vi "contour_levels_to_list.vi"(6 "Anchored Num":dbl, 7 "Mode":enum16{"Levels", "Intervals", "Level List"}(ring), 8 "Anchored at":bool, 9 "Min Max":T1, 10 "Levels/Int":sgl caption="Levels", 11 "Dimension":u16(ring) caption="Axis" items=["X", "Y", "Z"]) -> (3 "Item Names":string[](array[string]))   [LabVIEW 2020, in "3DPC_SurfacePlot.xctl"]
uses:
  <vilib>/Native 3D Graph/xcontrol/3DPC_SurfacePlot.xctl
  <vilib>/Native 3D Graph/typedefs/range_cluster.ctl
  <vilib>/Native 3D Graph/typedefs/min_max.ctl
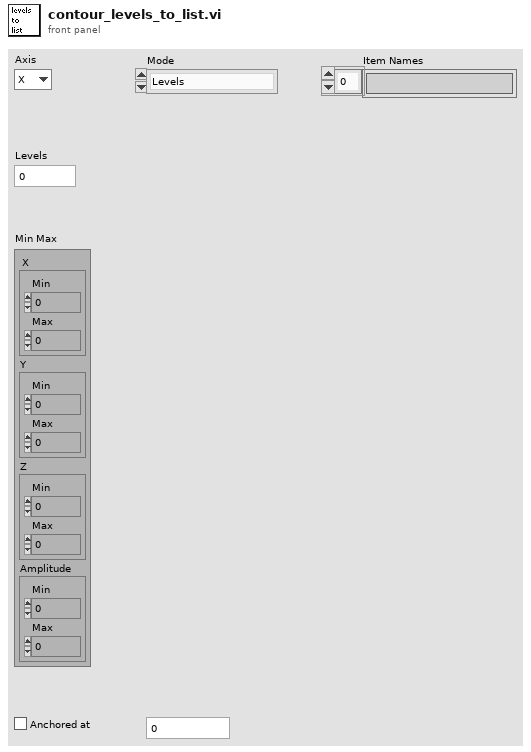
[diagram p1: front panel]
types:
  T1 = typedef "3DPC_SurfacePlot.xctl/range_cluster.ctl" = cluster{"X":T2, "Y":T2, "Z":T2, "Amplitude":T2}
  T2 = typedef "3DPC_SurfacePlot.xctl/min_max.ctl" = cluster{"Min":sgl, "Max":sgl}
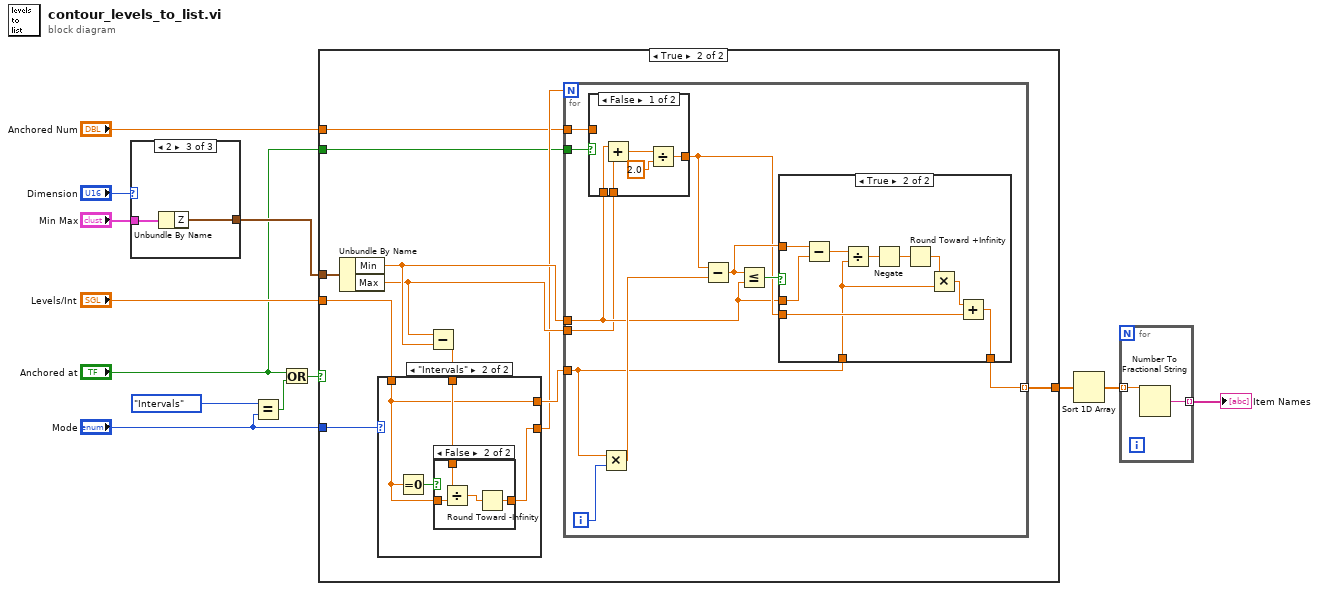
[diagram p0: block diagram]
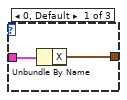
[diagram p2: hidden frame]
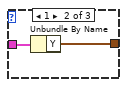
[diagram p3: hidden frame]
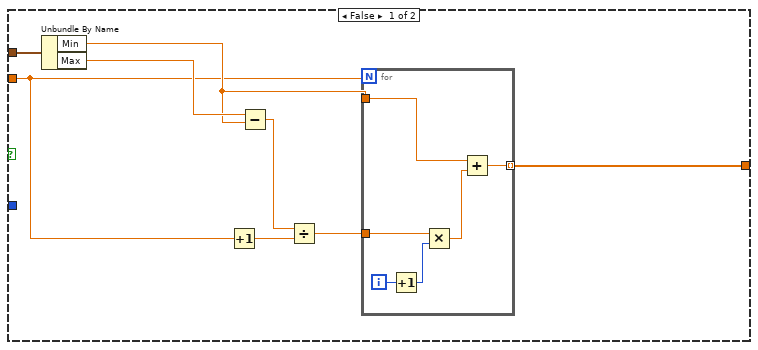
[diagram p4: hidden frame]
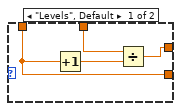
[diagram p5: hidden frame]
diagram:
  n1 = case shown="2" "Dimension" {
    tunnel: "Min Max" -> [w15 w17 w19]
    tunnel: [w14 w16 w18] -> w10
    frame 0, Default {
      n2 = Unbundle By Name(w15) -> ("X"=w14:T2)
    }
    frame 1 {
      n3 = Unbundle By Name(w17) -> ("Y"=w16:T2)
    }
    frame 2 {
      n4 = Unbundle By Name(w19) -> ("Z"=w18:T2)
    }
  }
  n5 = Equal?(x=enum16{"Levels", "Intervals", "Level List"}."Intervals" ("Mode"), y="Mode") -> (x = y?=w6:bool)
  n6 = Or(x="Anchored at", y=w6) -> (x .or. y?=w5:bool)
  n7 = case shown="True" w5 {
    tunnel: "Levels/Int" -> [w21 w40]
    tunnel: w10 -> [w27 w44]
    tunnel: [w22 w38] -> w8
    tunnel: "Mode" -> [_ w36]
    tunnel: "Anchored at" -> [_ w35]
    tunnel: "Anchored Num" -> [_ w34]
    frame False {
      n8 = Unbundle By Name(w27) -> ("Min"=w25:sgl, "Max"=w26:sgl)
      n9 = Increment(x=w21) -> (x+1=w20:sgl)
      n10 = Subtract(x=w26, y=w25) -> (x-y=w24:sgl)
      n11 = Divide(x=w24, y=w20) -> (x/y=w23:sgl)
      n12 = for {
        N: w21 -> [_]
        tunnel: w25 -> [w32]
        tunnel: w23 -> [w33]
        tunnel: [w28] -> w22 mode=indexing
        i -> [w30]
        n13 = Increment(x=w30) -> (x+1=w29:i32)
        n14 = Multiply(x=w33, y=w29) -> (x*y=w31:sgl)
        n15 = Add(x=w32, y=w31) -> (x+y=w28:sgl)
      }
    }
    frame True {
      n16 = Unbundle By Name(w44) -> ("Min"=w43:sgl, "Max"=w39:sgl)
      n17 = Subtract(x=w39, y=w43) -> (x-y=w42:sgl)
      n18 = case shown="\"Intervals\"" w36 {
        tunnel: w42 -> [w48 w52]
        tunnel: [w47 w50] -> w41
        tunnel: w40 -> [w45 w50]
        tunnel: [w45 w51] -> w37
        frame "Levels", Default {
          n19 = Increment(x=w45) -> (x+1=w46:sgl)
          n20 = Divide(x=w48, y=w46) -> (x/y=w47:sgl)
        }
        frame "Intervals" {
          n21 = Equal To 0?(x=w50) -> (x = 0?=w49:bool)
          n22 = case shown="False" w49 {
            tunnel: [w53 w54] -> w51
            tunnel: w52 -> [_ w56]
            tunnel: w50 -> [w53 w55]
            frame True {
            }
            frame False {
              n23 = Divide(x=w56, y=w55) -> (x/y=w57:sgl)
              n24 = Round Toward -Infinity(1:w57) -> (0:w54:sgl)
            }
          }
        }
      }
      n25 = for {
        N: w37 -> [_]
        tunnel: w43 -> [w61]
        tunnel: w41 -> [w64]
        tunnel: w39 -> [w60]
        tunnel: [w62] -> w38 mode=indexing
        tunnel: w35 -> [w59]
        tunnel: w34 -> [w58]
        i -> [w68]
        n26 = case shown="False" w59 {
          tunnel: [w69 w74] -> w63
          tunnel: w61 -> [w72 _]
          tunnel: w60 -> [w71 _]
          tunnel: w58 -> [_ w74]
          frame False {
            n27 = Add(x=w72, y=w71) -> (x+y=w70:sgl)
            n28 = Divide(x=w70, y=sgl 2.0) -> (x/y=w69:sgl)
          }
          frame True {
          }
        }
        n29 = Multiply(x=w64, y=w68) -> (x*y=w67:sgl)
        n30 = Subtract(x=w63, y=w67) -> (x-y=w65:dbl)
        n31 = Less Or Equal?(x=w65, y=w61) -> (x <= y?=w66:bool)
        n32 = case shown="True" w66 {
          tunnel: w65 -> [w75 w85]
          tunnel: [w75 w78] -> w62
          tunnel: w61 -> [_ w84]
          tunnel: w64 -> [_ w80]
          tunnel: w63 -> [_ w82]
          frame False {
          }
          frame True {
            n33 = Subtract(x=w85, y=w84) -> (x-y=w83:dbl)
            n34 = Divide(x=w83, y=w80) -> (x/y=w77:dbl)
            n35 = Negate(x=w77) -> (-x=w76:dbl)
            n36 = Round Toward +Infinity(x=w76) -> (ceil(x): smallest int >= x=w81:dbl)
            n37 = Multiply(x=w81, y=w80) -> (x*y=w79:dbl)
            n38 = Add(x=w79, y=w82) -> (x+y=w78:dbl)
          }
        }
      }
    }
  }
  n39 = Sort 1D Array(array=w8) -> (sorted array=w7:dbl[])
  n40 = for {
    tunnel: w7 -> [w87] mode=indexing
    tunnel: [w86] -> w9 mode=indexing
    n41 = Number To Fractional String(number=w87) -> (F-format string=w86:string)  [unwired: 3 out]
  }
  "Item Names" <- w9
